vi "Counter.vi"(10 "Counts Chart Refnum":refnum<vi>, 11 "Counts/s Ref":refnum<vi>) -> ()   [LabVIEW 2012]
uses:
  <vilib>/DAQmx/read.llb/DAQmx Read (Counter U32 1Chan 1Samp).vi
  Channels.vi
  <vilib>/DAQmx/create/channels.llb/DAQmx Create Channel (CI-Count Edges).vi
  Global Vars.vi
  <vilib>/DAQmx/miscellaneous.llb/DAQmx Fill In Error Info.vi
panel:
  out "Counts/s":i32
  out "Counts Chart":u32(graph)
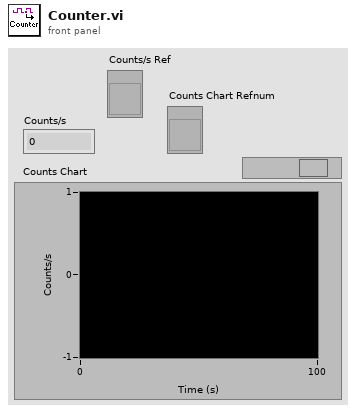
[diagram p1: front panel]
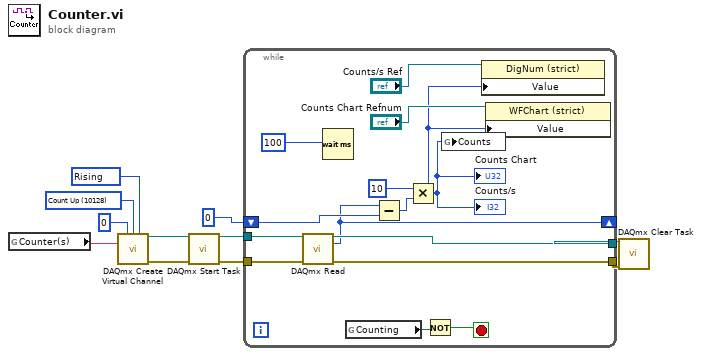
[diagram p0: block diagram]
diagram:
  w9 = 10280 items=["Rising"=10280, "Falling"=10171] ("Edge")
  w10 = 10128 items=["Count Up"=10128, "Count Down"=10124, "Externally Controlled"=10326] ("Count Direction")
  n1 = global read "Channels.vi" "Counter(s)"() -> (w8:tag)
  n2 = call-poly <vilib>:"DAQmx Create Virtual Channel.vi"("initial count"=u32 0 ("Initial Count"), "count direction"=w10, "edge"=w9, "counter"=w8) -> ("task out"=w7:refnum<k21>, "error out"=w6:errorcluster)  [unwired: 10 in]
  n3 = call <vilib>:"DAQmx Start Task.vi"("task/channels in"=w7, "error in"=w6) -> ("task out"=w5:refnum<k21>, "error out"=w4:errorcluster)  [unwired: 12 in]
  n4 = while {
    tunnel: w5 -> [w23]
    tunnel: w4 -> [w22]
    shift-right: [w17] -> _
    shift-left: 0 -> [w21]
    tunnel: [w19] -> w2
    tunnel: [w18] -> w1
    stop <- w24 stop-if-true
    n5 = call-poly <vilib>:"DAQmx Read.vi"("task/channels in"=w23, "error in"=w22) -> ("task out"=w19:refnum<k21>, "data"=w17:u32, "error out"=w18:errorcluster)  [unwired: 11 in]
    n6 = Wait (ms)(milliseconds to wait=100) -> ()  [unwired: 1 out]
    n7 = global read "Global Vars.vi" "Counting"() -> (w25:bool)
    n8 = Subtract(x=w17, y=w21) -> (x-y=w15:u32)
    n9 = Multiply(x=10, y=w15) -> (x*y=w12:u32)
    "Counts/s" <- w12
    "Counts Chart" <- w12
    n10 = Not(x=w25) -> (.not. x?=w24:bool)
    n11 = global write "Global Vars.vi" "Counts"(w12) -> ()
    n12 = property class="DigNum (strict)"(reference="Counts/s Ref", "Value"=w12) -> ()  [unwired: 1 in, 2 out]
    n13 = property class="WFChart (strict)"(reference="Counts Chart Refnum", "Value"=w12) -> ()  [unwired: 1 in, 2 out]
  }
  n14 = call <vilib>:"DAQmx Clear Task.vi"("task in"=w2, "error in"=w1) -> ()  [unwired: 13 in, 1 out]
